vi "Unsubscribe Topic.vi"(7 "Close if last?":bool, 8 "error in (no error)":errorcluster, 10 "Receivers Enqueuer":refnum<class "Message Enqueuer.lvclass">, 11 "Topic  (ALL)":string="*") -> (0 "error out":errorcluster)   [LabVIEW 2020, in "Actor Pub Sub Channels.lvlib"]
uses:
  Actor Pub Sub Channels.lvlib
  <vilib>/ActorFramework/Message Enqueuer/Message Enqueuer.lvclass
  Pub Sub Message Channel/Pub Sub Message Channel.lvclass
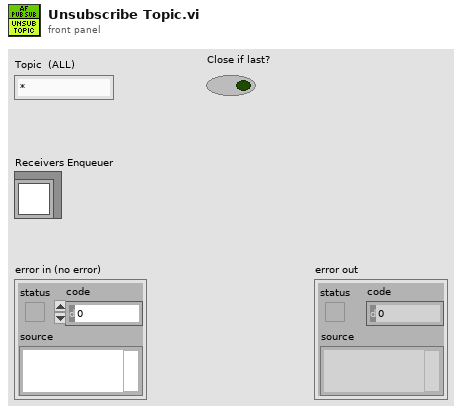
[diagram p1: front panel]
types:
  T1 = enum16{"Nothing", "Get Channel", "Get Or Create Channel", "Close Channel", "Dispose"}
  T2 = map{string, refnum<class "Pub Sub Message Channel.lvclass">}
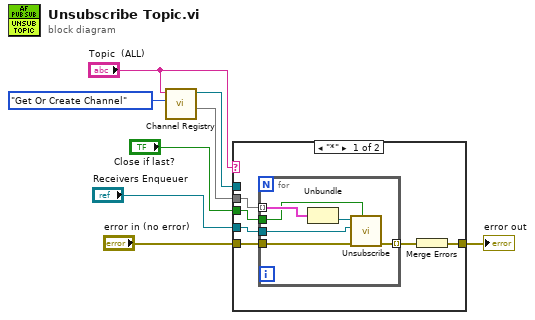
[diagram p0: block diagram]
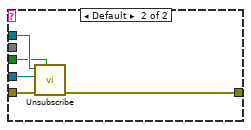
[diagram p2: hidden frame]
diagram:
  n1 = call "Channel Registry.vi"("Action"=T1."Get Or Create Channel", "Topic"="Topic  (ALL)") -> ("Registered Channels"=w1:T2, "Pub Sub Message Channel"=w7:refnum<class "Pub Sub Message Channel.lvclass">)  [unwired: 7 in, 1 out]
  n2 = case shown="\"*\"" "Topic  (ALL)" {
    tunnel: w7 -> [_ w25]
    tunnel: "Receivers Enqueuer" -> [w13 w24]
    tunnel: "error in (no error)" -> [w12 w23]
    tunnel: [w10 w22] -> w4
    tunnel: "Close if last?" -> [w9 w21]
    tunnel: w1 -> [w14 _]
    frame "*" {
      n3 = for {
        tunnel: w14 -> [w20] mode=indexing
        tunnel: w13 -> [w18]
        tunnel: w12 -> [w17]
        tunnel: [w16] -> w11 mode=indexing
        tunnel: w9 -> [w15]
        n4 = Unbundle(w20) -> ("Pub Sub Message Channel out"=w19:refnum<class "Pub Sub Message Channel.lvclass">)  [unwired: 1 out]
        n5 = call-dynamic "Unsubscribe.vi"("Close if last?"=w15, "error in (no error)"=w17, "Receivers Enqueuer"=w18, "Pub Sub Message Channel in"=w19) -> ("error out"=w16:errorcluster)  [unwired: 6 in, 1 out]
      }
      n6 = Merge Errors(w11) -> (w10:errorcluster)
    }
    frame Default {
      n7 = call-dynamic "Unsubscribe.vi"("Close if last?"=w21, "error in (no error)"=w23, "Receivers Enqueuer"=w24, "Pub Sub Message Channel in"=w25) -> ("error out"=w22:errorcluster)  [unwired: 6 in, 1 out]
    }
  }
  "error out" <- w4
